vi "nonIterativeImageStatistics.vi"(11 "HOL in":dbl[][][](array[numeric])) -> (1 "var n+1":dbl[][](array[numeric]), 2 "MU n+1":dbl[][](array[numeric]))   [LabVIEW 2018, in "statistics.lvlib"]
uses:
  statistics.lvlib
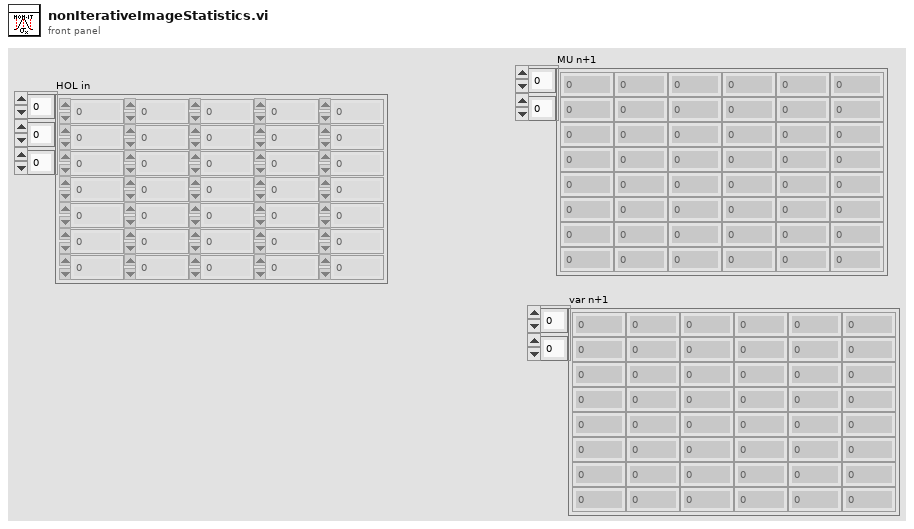
[diagram p1: front panel]
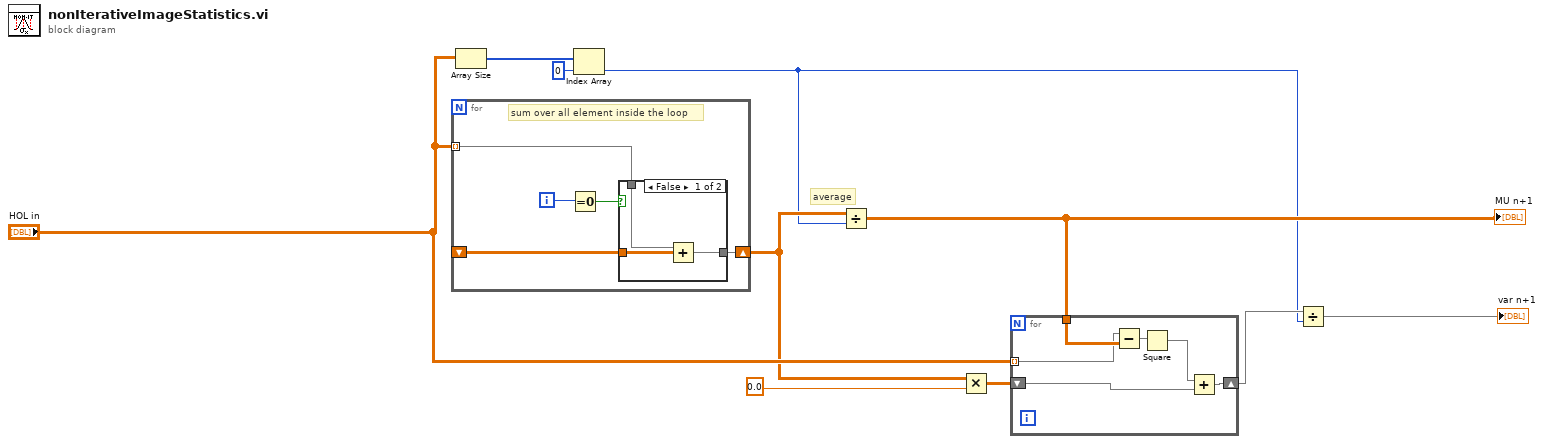
[diagram p0: block diagram]
diagram:
  # "average"
  n1 = for {
    shift-right: [w15] -> w5
    shift-left: _ -> [w14]
    tunnel: "HOL in" -> [w11] mode=indexing
    i -> [w12]
    # "sum over all element inside the loop"
    n2 = Equal To 0?(x=w12) -> (x = 0?=w13:bool)
    n3 = case shown="False" w13 {
      tunnel: w14 -> [w18 _]
      tunnel: [w17 w19] -> w15
      tunnel: w11 -> [w16 w19]
      frame False {
        n4 = Add(x=w16, y=w18) -> (x+y=w17:dbl[][])
      }
      frame True {
      }
    }
  }
  n5 = Array Size(array="HOL in") -> (size(s)=w3:i32[])
  n6 = Index Array(array=w3, index=0) -> (element=w1:i32)
  n7 = Divide(x=w5, y=w1) -> (x/y=w9:dbl[][])
  "MU n+1" <- w9
  n8 = Multiply(x=w5, y=0.0) -> (x*y=w6:dbl[][])
  n9 = for {
    shift-right: [w21] -> w7
    shift-left: w6 -> [w23]
    tunnel: w9 -> [w22]
    tunnel: "HOL in" -> [w20] mode=indexing
    n10 = Subtract(x=w20, y=w22) -> (x-y=w25:dbl[][])
    n11 = Square(x=w25) -> (x^2=w24:dbl[][])
    n12 = Add(x=w24, y=w23) -> (x+y=w21:dbl[][])
  }
  n13 = Divide(x=w7, y=w1) -> (x/y=→"var n+1":dbl[][])
